vi "test Verify AND Combos.vi"(8 "error in":errorcluster, 11 "Test Case In":refnum<class "LUnit Extensions Tests.lvclass">) -> (0 "error out":errorcluster, 3 "Test Case Out":refnum<class "LUnit Extensions Tests.lvclass">)   [LabVIEW 2020, in "LUnit Extensions Tests.lvclass"]
uses:
  LUnit Extensions Tests.lvclass
  C:/Program Files/National Instruments/LabVIEW 2026/vi.lib/Astemes/LUnit/Test Case.lvclass
  a51d05ad-22a6-4aae-b852-1cd07aba18e9.vi
  Source/Extensions/LUnit.Extension/LUnit.Extension.lvlib
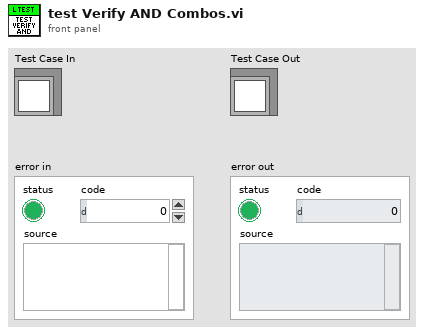
[diagram p1: front panel]
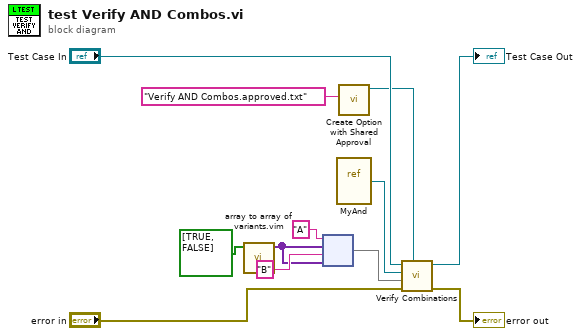
[diagram p0: block diagram]
diagram:
  n1 = call "array to array of variants.vim"("Array in"=bool[] [TRUE, FALSE]) -> ("Array out"=w5:variant[])  [unwired: 10 in]
  n2 = node ("Build Map")("A" ("key"), w5, "B" ("key"), w5) -> (w3:map{string, variant[]})
  n3 = vi-ref "MyAnd.vi"() -> (w4:refnum<vi>)
  n4 = call "Create Option with Shared Approval.vi"("Filename"="Verify AND Combos.approved.txt") -> ("Options outs"=w1:refnum<class "Options.lvclass">)  [unwired: 10 in]
  n5 = call "Verify Combinations.vi"("Options"=w1, "error in"="error in", "ctl label -> value var[]"=w3, "VI in"=w4, "LUnit Test Case In"="Test Case In") -> ("error out"=→"error out":errorcluster, "LUnit Test Case Out"=→"Test Case Out":refnum<class "LUnit Extensions Tests.lvclass">)  [unwired: 5 in]
